vi "Destroy Client.vi"(8 "error in":errorcluster, 11 "gRPC ID":T1) -> (0 "error out":errorcluster)   [LabVIEW 2021, in "CIFPluginLoaderClientWrapper.lvlib"]
uses:
  CIFPluginLoaderClientWrapper.lvlib
  <vilib>/gRPC/LabVIEW gRPC Library/grpc-lvsupport-release.lvlib
  <vilib>/gRPC/LabVIEW gRPC Library/Shared/grpcId.ctl
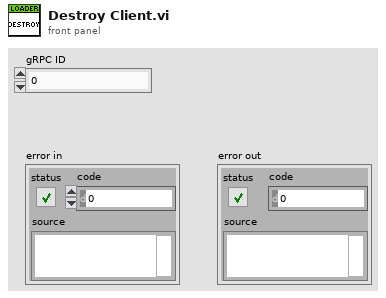
[diagram p1: front panel]
types:
  T1 = typedef "grpc-lvsupport-release.lvlib/grpcId.ctl" = u64
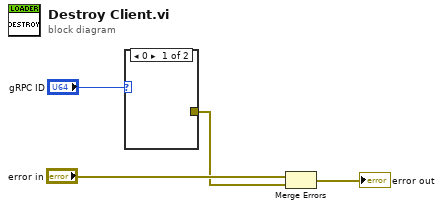
[diagram p0: block diagram]
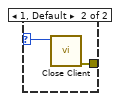
[diagram p2: hidden frame]
diagram:
  n1 = case shown="0" "gRPC ID" {
    selector: "gRPC ID" -> [_ w5]
    tunnel: [_ w6] -> w2
    frame 0 {
    }
    frame 1, Default {
      n2 = call <vilib>:"Close Client.vi"("ClientID in"=w5) -> ("error out"=w6:errorcluster)  [unwired: 10 in]
    }
  }
  n3 = Merge Errors("error in", w2) -> (→"error out":errorcluster)
